vi "read_data_with_TCP.vi"(8 "error_in":errorcluster, 11 "TCP_ref_in":refnum<k5>) -> (0 "error_out":errorcluster, 2 "data_out":dbl[](array[numeric]), 3 "TCP_ref_out":refnum<k5>)   [LabVIEW 2024]
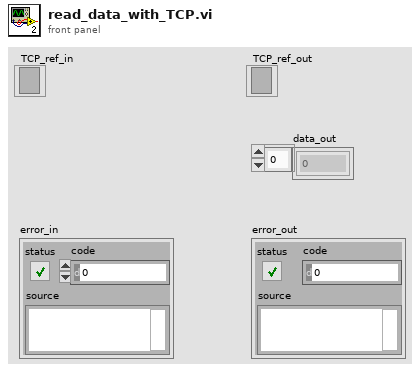
[diagram p1: front panel]
types:
  T1 = enum16{"Standard", "Buffered", "CRLF", "Immediate"}
  T2 = enum16{"big-endian, network order", "native, host order", "little-endian"}
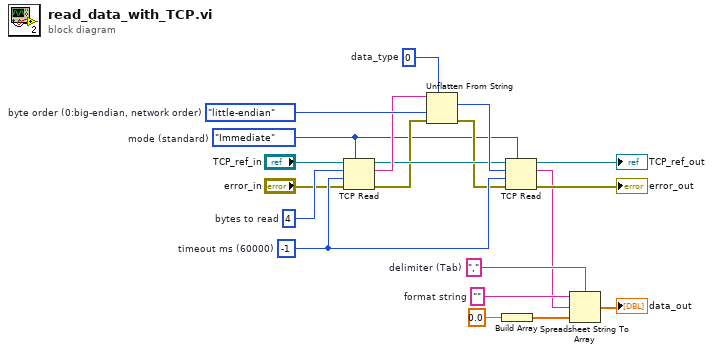
[diagram p0: block diagram]
diagram:
  w1 = T1."Immediate"  # mode (standard)
  w16 = -1  # timeout ms (60000)
  w20 = T2."little-endian"  # byte order (0:big-endian, network order)
  w18 = 0  # data_type
  w15 = 4  # bytes to read
  w8 = ","  # delimiter (Tab)
  w7 = ""  # format string
  n1 = TCP Read(connection ID="TCP_ref_in", bytes to read=w15, error in (no error)="error_in", 7:w1, 9:w16) -> (connection ID out=w13:refnum<k5>, data out=w17:string, error out=w3:errorcluster)
  n2 = Unflatten From String(type=w18, binary string=w17, byte order (0:big-endian, network order)=w20, error in (no error)=w3) -> (value=w19:i32, error out=w2:errorcluster)  [unwired: 1 in, 1 out]
  n3 = Build Array(0.0) -> (w5:dbl[])
  n4 = TCP Read(connection ID=w13, bytes to read=w19, error in (no error)=w2, 7:w1, 9:w16) -> (connection ID out=→"TCP_ref_out":refnum<k5>, data out=w6:string, error out=→"error_out":errorcluster)
  n5 = Spreadsheet String To Array(delimiter (Tab)=w8, format string=w7, spreadsheet string=w6, array type (2D Dbl)=w5) -> (array=→"data_out":dbl[])
